vi "LockinRemoteControl.setREFconfig.vi"(8 "error in (no error)":errorcluster, 10 "setREFconfig":T1={"Channels: Lockin"={"REF f (Hz)"=[13.0], "REF phi (°)"=[0.0, 0.0, 0.0, 0.0, 0.0, 0.0, 0.0, 0.0]}} {"Channels: Lockin"."REF phi (°)" format="%#_3g"}, 11 "RemoteControl":refnum<class "LockinRemoteControl.lvclass">) -> (0 "error out":errorcluster, 3 "RemoteControl out":refnum<class "LockinRemoteControl.lvclass">)   [LabVIEW 2016, in "LockinRemoteControl.lvclass"]
doc: "---------------------------------------------------------------\nJKI State Machine Objects™\nhttp://jki.net/state-machine-objects/\nCopyright (C) 2005-2015, JKI <info@jki.net>\nALL RIGHTS RESERVEDJKI State Machine Objects (SMO) 1.0.0.4\nJKI - JKI\nCopyright (c) 2015, JKI"
uses:
  LockinRemoteControl.lvclass
  Typedefs/PrivateEvents--LockinRemoteControl.setREFconfig.ctl
  Typedefs/REF-cluster.ctl
  Typedefs/REF_f-array.ctl
  Typedefs/REF_phi-array.ctl
  LockinRemoteControl.lvclass/LockinRemoteControl.ctl
panel:
  # "For instructions on how to use the JKI State Machine Objects, examples and video tutorials, visit:\nhttp://jki.net/state-machine-objects/\n\nJKI State Machine Objects™\nhttp://jki.net/state-machine-objects/\nCopyright (C) 2005-2015, JKI <info@jki.net>\nALL RIGHTS RESERVED"
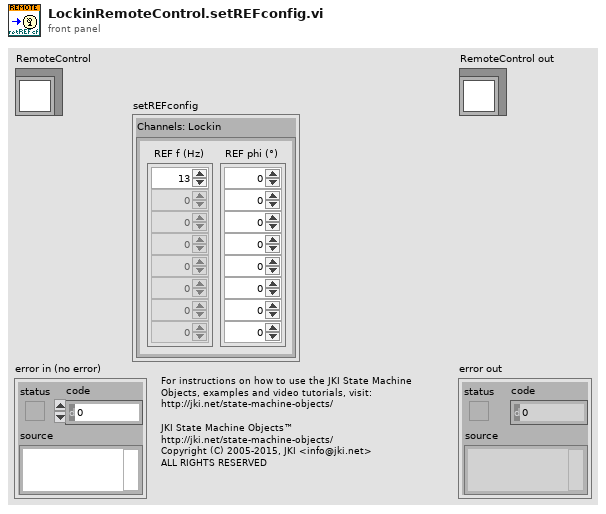
[diagram p1: front panel]
types:
  T1 = typedef "LockinRemoteControl.lvclass/PrivateEvents--LockinRemoteControl.setREFconfig.ctl" = cluster{"Channels: Lockin":T2}
  T2 = typedef "REF-cluster.ctl" = cluster{"REF f (Hz)":T3, "REF phi (°)":T4}
  T3 = typedef "REF_f-array.ctl" = dbl[]
  T4 = typedef "REF_phi-array.ctl" = dbl[]
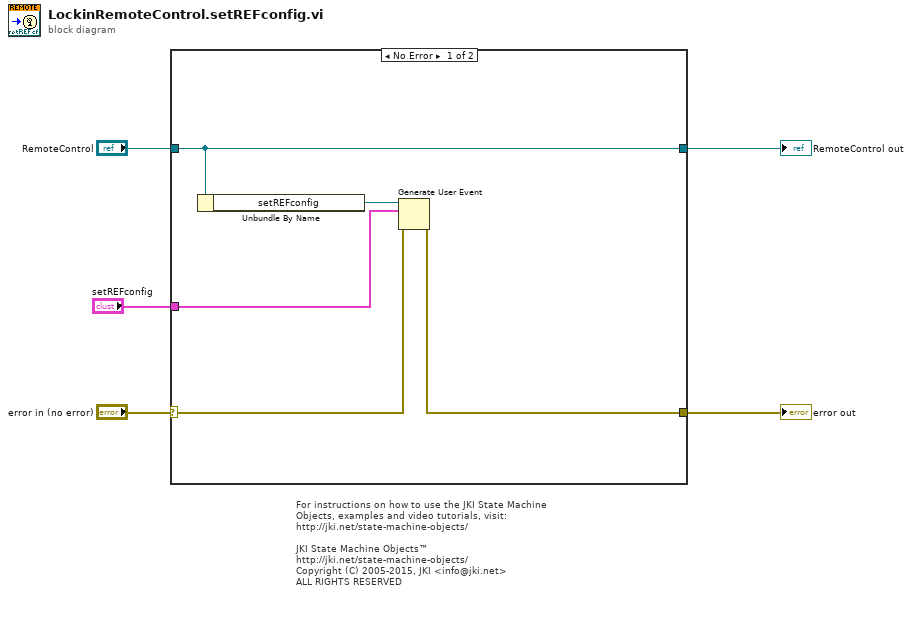
[diagram p0: block diagram]
diagram:
  # "For instructions on how to use the JKI State Machine Objects, examples and video tutorials, visit:\nhttp://jki.net/state-machine-objects/\n\nJKI State Machine Objects™\nhttp://jki.net/state-machine-objects/\nCopyright (C) 2005-2015, JKI <info@jki.net>\nALL RIGHTS RESERVED"
  n1 = case shown="No Error" "error in (no error)" {
    selector: "error in (no error)" -> [w10 w12]
    tunnel: [w7 w12] -> w4
    tunnel: [w6 w11] -> w5
    tunnel: "RemoteControl" -> [w6 w11]
    tunnel: "setREFconfig" -> [w9 _]
    frame No Error {
      n2 = Unbundle By Name(w6) -> ("setREFconfig"=w8:refnum<user-event>)
      n3 = Generate User Event(user event=w8, event data cluster=w9, error in=w10) -> (error out=w7:errorcluster)  [unwired: 1 in, 1 out]
    }
    frame Error {
    }
  }
  "error out" <- w4
  "RemoteControl out" <- w5
